vi "WaveOutput.vi"(0 "InitialValue":dbl, 1 "Max":dbl, 4 "Min":dbl, 5 "Increment":dbl=0.05 format="%#_13g") -> (7 "ValueOut":dbl)   [LabVIEW 2016]
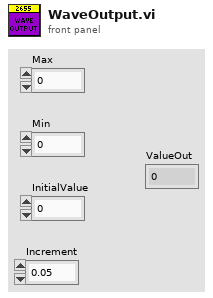
[diagram p1: front panel]
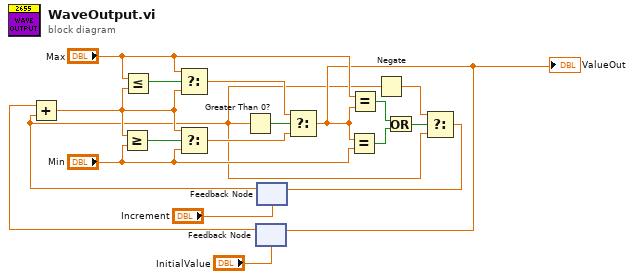
[diagram p0: block diagram]
diagram:
  n1 = feedback #1("InitialValue") -> (w5:dbl)
  n2 = feedback #2("Increment") -> (w3:dbl)
  n3 = Add(x=w5, y=w3) -> (x+y=w16:dbl)
  n4 = Greater Or Equal?(x=w16, y="Min") -> (x >= y?=w17:bool)
  n5 = Less Or Equal?(x="Max", y=w16) -> (x <= y?=w18:bool)
  n6 = Select(t="Max", s=w18, f=w16) -> (s? t:f=w14:dbl)
  n7 = Select(t=w16, s=w17, f="Min") -> (s? t:f=w13:dbl)
  n8 = Greater Than 0?(x=w3) -> (x > 0?=w15:bool)
  n9 = Select(t=w14, s=w15, f=w13) -> (s? t:f=w6:dbl)
  "ValueOut" <- w6
  n10 = feedback-in #1(w6) -> ()
  n11 = Equal?(x=w6, y="Min") -> (x = y?=w8:bool)
  n12 = Equal?(x="Max", y=w6) -> (x = y?=w9:bool)
  n13 = Negate(x=w3) -> (-x=w7:dbl)
  n14 = Or(x=w9, y=w8) -> (x .or. y?=w10:bool)
  n15 = Select(t=w7, s=w10, f=w3) -> (s? t:f=w4:dbl)
  n16 = feedback-in #2(w4) -> ()
